vi "JogContinuous.vi"(8 "error in (no error)":errorcluster, 10 "direction":i32(ring)=1 items=["Forward"=1, "Backward"=2], 11 "ThorlabsLabJack in":refnum<class "ThorlabsLabJack.lvclass">) -> (0 "error out":errorcluster, 3 "ThorlabsLabJack out":refnum<class "ThorlabsLabJack.lvclass">)   [LabVIEW 2018, in "ThorlabsLabJack.lvlib" / "ThorlabsLabJack.lvclass"]
uses:
  ThorlabsLabJack.lvclass
  ThorlabsLabJack.lvclass/ThorlabsLabJack.ctl
  C:/Projects/LabVIEW/In-Progress/Chetan Malpure/Axis/Thorlabs LabJack/Drivers/Thorlabs.MotionControl.IntegratedStepperMotorsCLI.dll
  Drivers/Thorlabs.MotionControl.IntegratedStepperMotorsCLI.dll
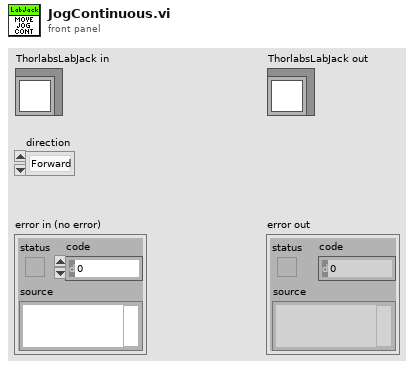
[diagram p1: front panel]
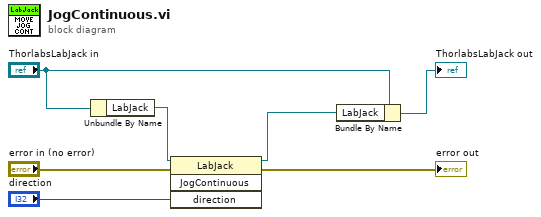
[diagram p0: block diagram]
diagram:
  n1 = Unbundle By Name("ThorlabsLabJack in") -> ("LabJack"=w6:refnum<k24>)
  n2 = invoke class="LabJack" method="JogContinuous"(reference=w6, error in="error in (no error)", "direction"="direction") -> (reference out=w4:refnum<k24>, error out=→"error out":errorcluster)  [unwired: 1 in, 2 out]
  n3 = Bundle By Name(cluster="ThorlabsLabJack in", "LabJack"=w4) -> (→"ThorlabsLabJack out":refnum<class "ThorlabsLabJack.lvclass">)
